vi "Filter by Favorites.vi"(8 "error in (no error)":errorcluster, 10 "Favorites? (T)":bool=TRUE, 11 "Contacts":T1[](array[typedef])) -> (0 "error out":errorcluster, 3 "Filtered Contacts":T1[](array[typedef]))   [LabVIEW 2014, in "Map Data.lvlib"]
doc: "Filters an array of contacts to only include favorites or to not include favorites."
uses:
  Map Data.lvlib
  Control Sort Mode.ctl
  MapDatas.ctl
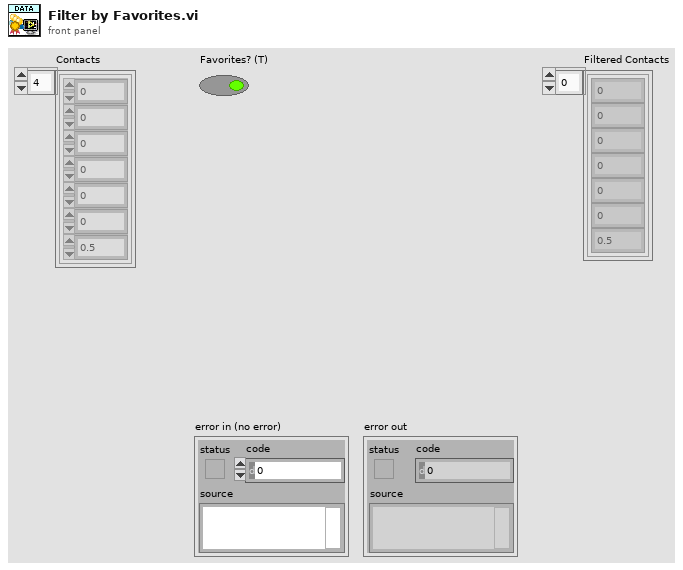
[diagram p1: front panel]
types:
  T1 = typedef "Map Data.lvlib/MapDatas.ctl" = cluster{"X":dbl, "Y":dbl, "Z":dbl, "heading":dbl, "X2":dbl, "Y2":dbl, "Z2":dbl}
  T2 = typedef "Map Data.lvlib/Control Sort Mode.ctl" = u16
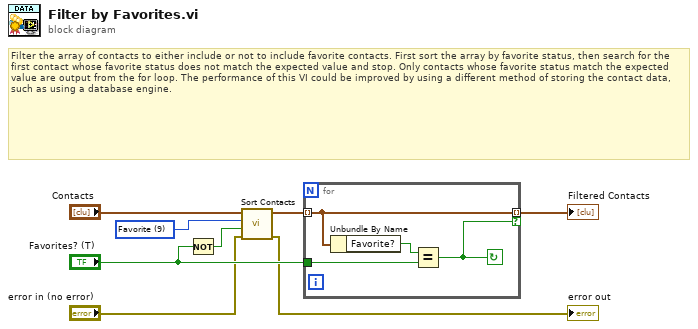
[diagram p0: block diagram]
diagram:
  w7 = T2 9 items=["Default", "Last Name", "First Name", "Middle Name", "Phone", "Street", "City", "State", "Postal Code", "Favorite"] ("Sort Mode (Default)")
  # "Filter the array of contacts to either include or not to include favorite contacts. First sort the array by favorite status, then search for the first contact whose favorite status does not match the expected value and stop. Only contacts whose favorite status match the expected value are output from the for loop. The performance of this VI could be improved by using a different method of storing the contact data, such as using a database engine."
  n1 = Not(x="Favorites? (T)") -> (.not. x?=w1:bool)
  n2 = call "Sort Contacts.vi"("error in (no error)"="error in (no error)", "Ascending? (T)"=w1, "Sort Mode (Default)"=w7, "Contacts"="Contacts") -> ("error out"=→"error out":errorcluster, "Sorted Contacts"=w4:T1[])  [unwired: 6 in]
  n3 = for {
    tunnel: w4 -> [w10] mode=indexing
    tunnel: "Favorites? (T)" -> [w11]
    tunnel: [w10] -> w2 mode=indexing if=w9
    stop <- w9 continue-if-true
    n4 = Unbundle By Name(w10) -> ("Favorite?"=w12:bool)
    n5 = Equal?(x=w12, y=w11) -> (x = y?=w9:bool)
  }
  "Filtered Contacts" <- w2
